vi "DHT11_labview_srednia_symulacja_stop.vi"() -> ()   [LabVIEW 2025]
uses:
  <vilib>/Utility/error.llb/Trim Whitespace One-Sided.vi
panel:
  out "numeric - start/stop":dbl
  in  "START/STOP":bool
  out "Temperatura œrednia[C]":dbl
  out "Wilgotnoœæ œrednia[%]":dbl
  out "Temperatura min[C]":dbl
  out "Temperatura max [C]":dbl
  out "Wilogtnoœæ min [%]":dbl
  out "Wilgotnosc max [%]":dbl
  out "Numeric iteracja while":i32
  out "wilgotnoœæ liczba":dbl
  out "Wilgotnoœæ wykres":dbl(graph)
  out "Temperatura liczba":dbl
  out "Temperatura wykres":dbl(graph)
  out "wyœwietlanie danych":string
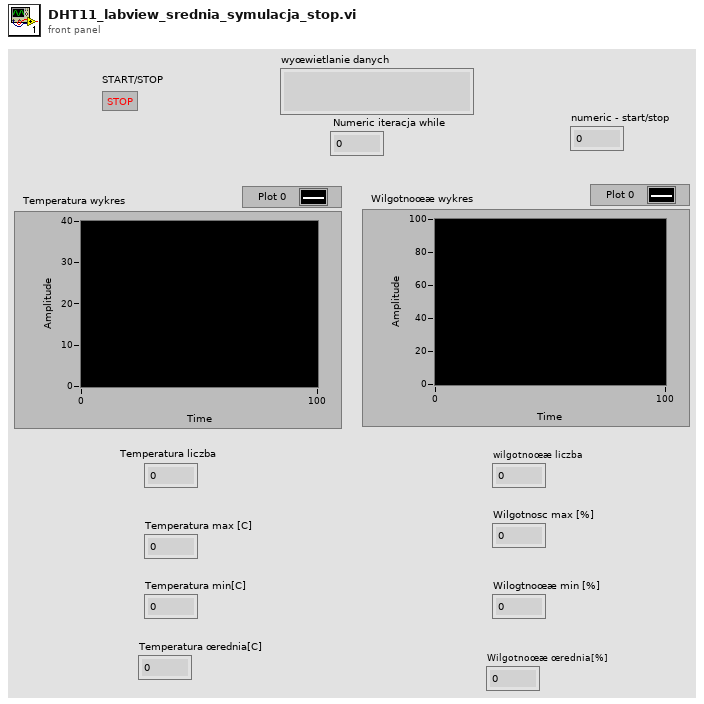
[diagram p1: front panel]
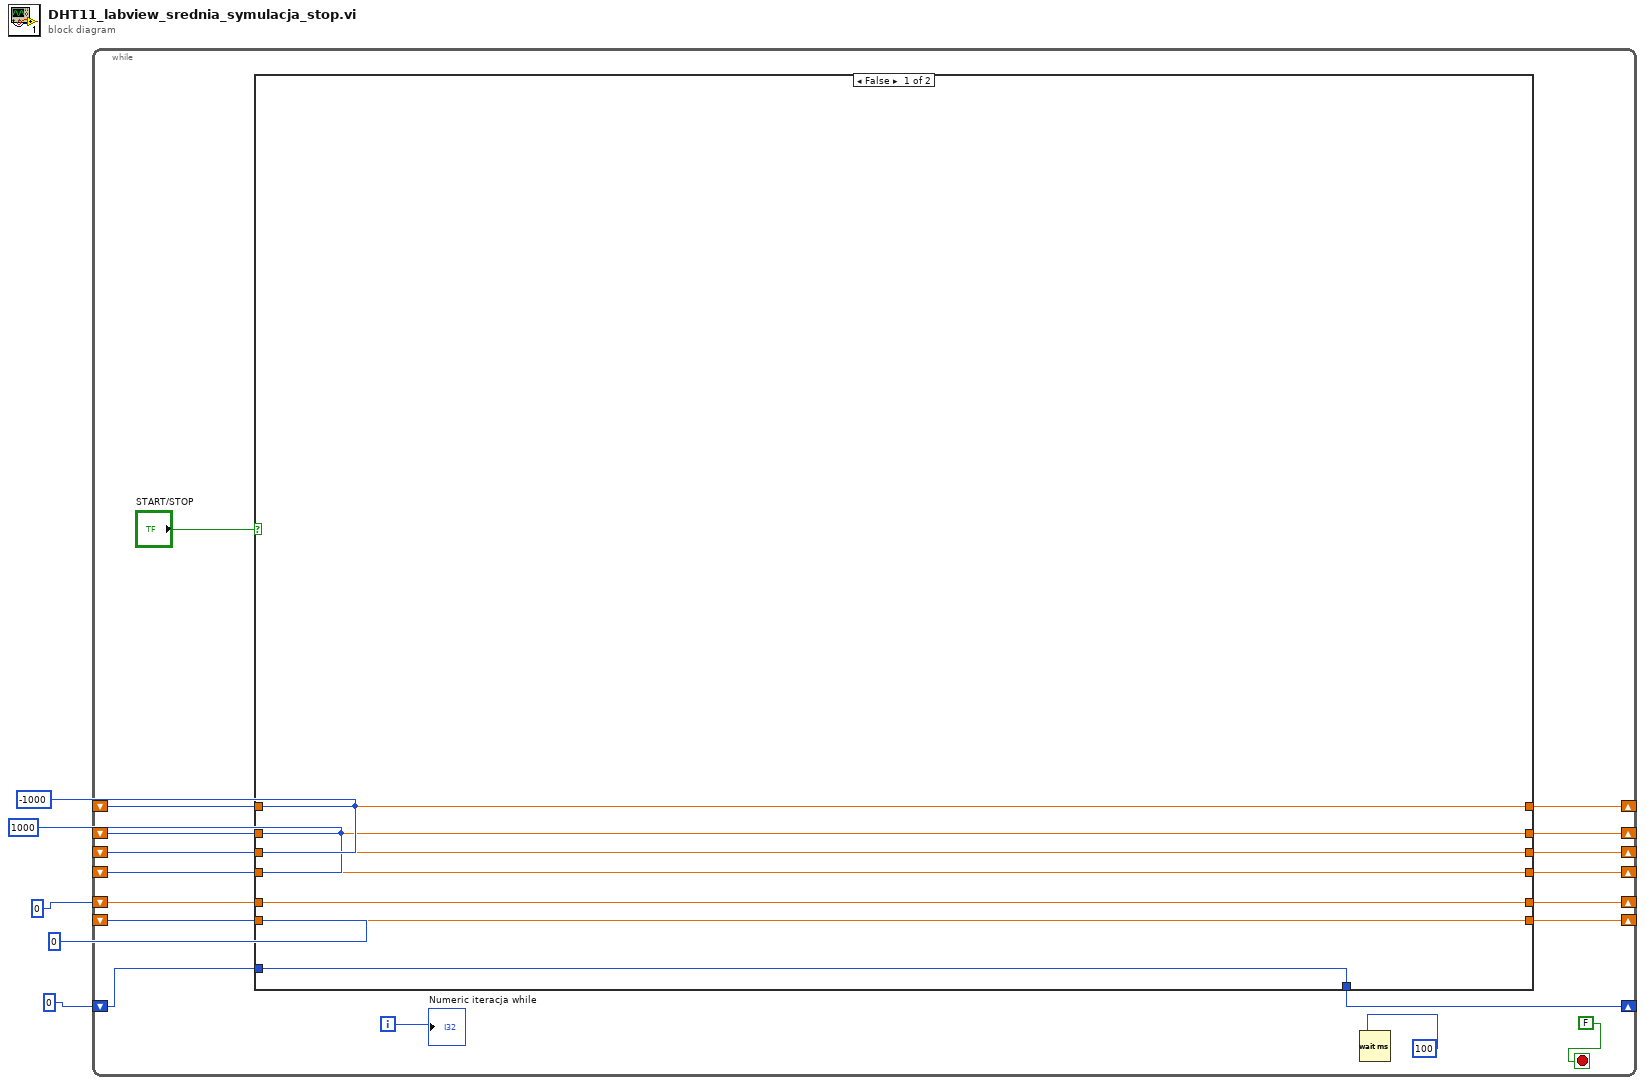
[diagram p0: block diagram]
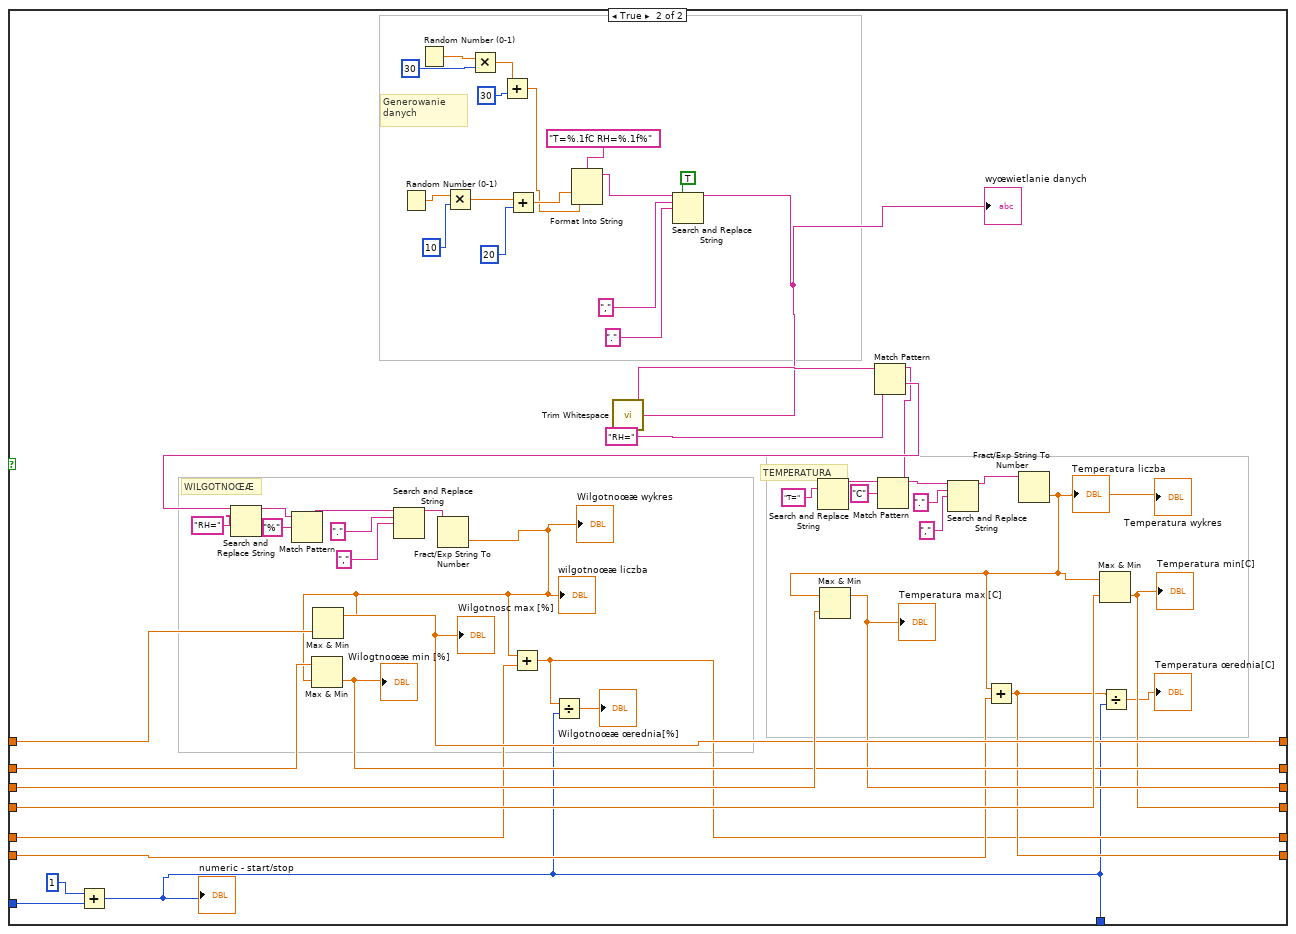
[diagram p2: hidden frame]
diagram:
  w4 = 1000
  w5 = -1000
  n1 = while {
    shift-right: [w18] -> _
    shift-left: w5 -> [w22]
    shift-right: [w17] -> _
    shift-left: w4 -> [w21]
    shift-right: [w16] -> _
    shift-left: w5 -> [w20]
    shift-right: [w15] -> _
    shift-left: w4 -> [w19]
    shift-right: [w11] -> _
    shift-left: 0 -> [w14]
    shift-right: [w12] -> _
    shift-left: 0 -> [w13]
    shift-right: [w7] -> _
    shift-left: 0 -> [w8]
    i -> [w10]
    stop <- FALSE stop-if-true
    n2 = case shown="False" "START/STOP" {
      tunnel: w22 -> [w29 w49]
      tunnel: w21 -> [w28 w48]
      tunnel: w20 -> [w27 w47]
      tunnel: w19 -> [w26 w46]
      tunnel: [w29 w45] -> w18
      tunnel: [w28 w44] -> w17
      tunnel: [w27 w43] -> w16
      tunnel: [w26 w42] -> w15
      tunnel: w14 -> [w25 w41]
      tunnel: w13 -> [w24 w38]
      tunnel: [w24 w36] -> w12
      tunnel: [w25 w34] -> w11
      tunnel: w8 -> [w30 w33]
      tunnel: [w30 w31] -> w7
      frame False {
      }
      frame True {
        # "Generowanie danych"
        # "WILGOTNOŒÆ"
        # "TEMPERATURA"
        n3 = Add(x=1, y=w33) -> (x+y=w31:i32)
        "numeric - start/stop" <- w31
        n4 = Random Number (0-1)() -> (number: 0 to 1=w62:dbl)
        n5 = Random Number (0-1)() -> (number: 0 to 1=w64:dbl)
        n6 = Multiply(x=w62, y=10) -> (x*y=w63:dbl)
        n7 = Multiply(x=w64, y=30) -> (x*y=w65:dbl)
        n8 = Add(x=w65, y=30) -> (x+y=w50:dbl)
        n9 = Add(x=w63, y=20) -> (x+y=w51:dbl)
        n10 = Format Into String(format string="T=%.1fC RH=%.1f%", w51, w50) -> (resulting string=w52:string)  [unwired: 2 in, 1 out]
        n11 = Search and Replace String(replace all?=TRUE, input string=w52, search string=",", replace string=".") -> (result string=w54:string)  [unwired: 4 in, 3 out]
        "wyœwietlanie danych" <- w54
        n12 = call <vilib>:"Trim Whitespace.vi"("string"=w54) -> ("trimmed string"=w75:string)  [unwired: 1 in]
        n13 = Match Pattern(string=w75, regular expression="RH=") -> (before substring=w76:string, after substring=w80:string)  [unwired: 1 in, 2 out]
        n14 = Search and Replace String(input string=w80, search string="RH=") -> (result string=w81:string)  [unwired: 6 in, 3 out]
        n15 = Match Pattern(string=w81, regular expression="%") -> (before substring=w82:string)  [unwired: 1 in, 3 out]
        n16 = Search and Replace String(input string=w82, search string=".", replace string="," ("replace string (\"\")")) -> (result string=w83:string)  [unwired: 5 in, 3 out]
        n17 = Fract/Exp String To Number(string=w83) -> (number=w40:dbl)  [unwired: 3 in, 1 out]
        "Wilgotnoœæ wykres" <- w40
        "wilgotnoœæ liczba" <- w40
        n18 = Max & Min(x=w48, y=w40) -> (min(x,y)=w44:dbl)  [unwired: 1 out]
        "Wilogtnoœæ min [%]" <- w44
        n19 = Max & Min(x=w40, y=w49) -> (max(x,y)=w45:dbl)  [unwired: 1 out]
        "Wilgotnosc max [%]" <- w45
        n20 = Add(x=w40, y=w41) -> (x+y=w34:dbl)
        n21 = Divide(x=w34, y=w31) -> (x/y=→"Wilgotnoœæ œrednia[%]":dbl)
        n22 = Search and Replace String(input string=w76, search string="T=" ("replace string (\"\")")) -> (result string=w77:string)  [unwired: 6 in, 3 out]
        n23 = Match Pattern(string=w77, regular expression="C") -> (before substring=w78:string)  [unwired: 1 in, 3 out]
        n24 = Search and Replace String(input string=w78, search string=".", replace string="," ("replace string (\"\")")) -> (result string=w79:string)  [unwired: 5 in, 3 out]
        n25 = Fract/Exp String To Number(string=w79) -> (number=w39:dbl)  [unwired: 3 in, 1 out]
        "Temperatura wykres" <- w39
        "Temperatura liczba" <- w39
        n26 = Max & Min(x=w39, y=w47) -> (max(x,y)=w43:dbl)  [unwired: 1 out]
        "Temperatura max [C]" <- w43
        n27 = Add(x=w39, y=w38) -> (x+y=w36:dbl)
        n28 = Max & Min(x=w39, y=w46) -> (min(x,y)=w42:dbl)  [unwired: 1 out]
        "Temperatura min[C]" <- w42
        n29 = Divide(x=w36, y=w31) -> (x/y=→"Temperatura œrednia[C]":dbl)
      }
    }
    n30 = Wait (ms)(milliseconds to wait=u32 100) -> ()  [unwired: 1 out]
    "Numeric iteracja while" <- w10
  }
